vi "TX data interpolation to DRAM.vi"() -> ()   [LabVIEW 2019]
uses:
  SubVIs/DRAM burst sequencer/Burst memo.ctl
  SubVIs/DRAM burst sequencer/DRAM mode.ctl
  SubVIs/DRAM burst sequencer/SegementSequencer_class/FPGA sequencer states.ctl
  <vilib>/Platform/TimedLoop/XDataNode/timing_clust.ctl
  <vilib>/Platform/TimedLoop/XDataNode/nitl_modes.ctl
  <vilib>/Platform/TimedLoop/XDataNode/wakeup.ctl
  SubVIs/DRAM burst sequencer/DRAM resources.ctl
  <instrlib>/_niInstr/Memory/v1/FPGA/DRAM U512/niInstr Memory DRAM U512 v1 FPGA.lvclass
  <instrlib>/_niInstr/Memory/v1/FPGA/BRAM U512/niInstr Memory BRAM U512 v1 FPGA.lvclass
  <instrlib>/_niInstr/Memory/v1/FPGA/DRAM U512/Public/Create.vi
  <instrlib>/_niInstr/Memory/v1/FPGA/BRAM U512/Public/Create.vi
  <vilib>/rvi/DataTransferAndStorage/Container/Common/niFpgaContainerGetUniqueNameForEmu.vi
  <vilib>/rvi/DataTransferAndStorage/Container/Common/niFpgaContainerSetEmuInfo.vi
  <vilib>/rvi/eio/common/nirviEmuReportErrorAndStop.vi
  <vilib>/rvi/Emulation/niFpgaSctlEmulationGetInTimedLoop.vi
  <vilib>/rvi/Emulation/niFpgaEmulationReportErrorSimple.vi
  <vilib>/rvi/Emulation/niFpgaGetClockAttributes.vi
  <vilib>/rvi/Emulation/niFpgaCriticalErrorInLSC.vi
  <vilib>/rvi/Emulation/niFpgaProcessEmulError.vi
  <vilib>/Platform/TimedLoop/XDataNode/XDataNode.xnode
  <vilib>/rvi/LocalResourceManager/LocalResourceManager.xnode
  SubVIs/DRAM burst sequencer/SegementSequencer_class/SegmentSequencer.lvclass
  <instrlib>/_niInstr/Memory/v1/FPGA/DRAM/niInstr Memory DRAM v1 FPGA.lvclass
  <vilib>/Platform/TimedLoop/XDataNode/XDNodeRunTimeDep.lvlib
  SubVIs/DRAM burst sequencer/TX burst sequencer.lvlib
  <instrlib>/_niInstr/Basic Elements/v1/FPGA/niInstr Basic Elements v1 FPGA.lvlib
  <instrlib>/_niInstr/Memory/v1/FPGA/BRAM/niInstr Memory BRAM v1 FPGA.lvclass
panel:
  out "bram.debug ctr":T1
  out "bram.last written addr":u32
  in  "seq.start":bool
  in  "seq.rst":bool
  out "seq.state":T2
  out "seq.step ctr":u32
  out "seq.repeat ctr":u64
  out "seq.loaded steps":u32
  out "seq.req ctr":i64
  in  "seq.continous":bool
  in  "seq.add step":bool
  in  "seq.new step":T3
  in  "memo.reset":bool
  in  "memo.ctr rst":bool
  out "dram.last written addr":u32
  out "dram.debug ctr":T1
  in  "memo mode":T4
  out "flush":bool
  in  "iq.load":bool
  in  "iq.load addr":u32
  in  "burst memo":T5
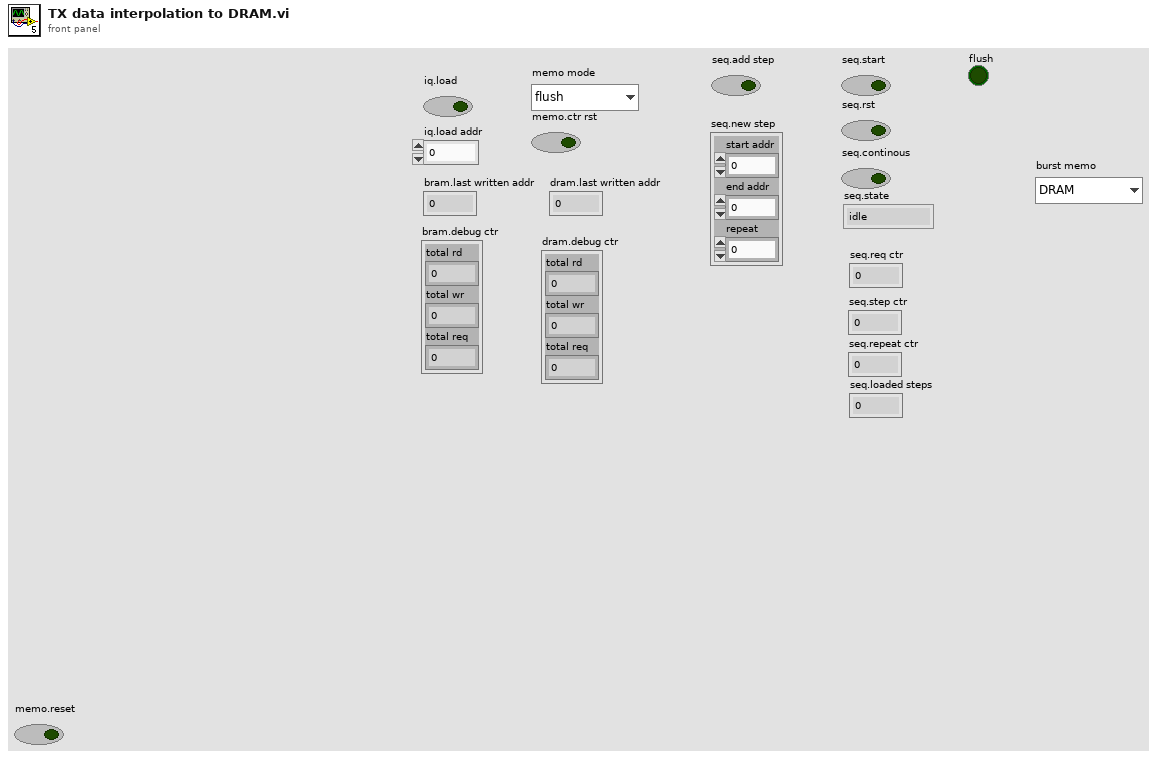
[diagram p1: front panel]
types:
  T1 = cluster{"total rd":u32, "total wr":u32, "total req":u32}
  T2 = typedef "FPGA sequencer states.ctl" = enum16{"idle", "read step", "execute step"}
  T3 = cluster{"start addr":u32, "end addr":u32, "repeat":u64}
  T4 = typedef "TX burst sequencer.lvlib/DRAM mode.ctl" = enum16{"flush", "reset", "write", "read"}
  T5 = typedef "TX burst sequencer.lvlib/Burst memo.ctl" = enum16{"DRAM", "BRAM"}
  T6 = typedef "TX burst sequencer.lvlib/DRAM resources.ctl" = cluster{"DRAM read data FIFO":refnum<k21>, "DRAM write data FIFO":refnum<k21>, "DRAM request FIFO":refnum<k21>, "DRAM U512 memo":refnum<class "niInstr Memory DRAM U512 v1 FPGA.lvclass">, "DMA data loader":refnum<k21>, "BRAM read data FIFO":refnum<k21>, "BRAM write data FIFO":refnum<k21>, "BRAM request FIFO":refnum<k21>, "BRAM U512 memo":refnum<class "niInstr Memory BRAM U512 v1 FPGA.lvclass">}
  T7 = typedef "XDNodeRunTimeDep.lvlib/timing_clust.ctl" = cluster{"Expected End [f-1]":u64, "Actual End [f-1]":u64, "Finished Late? [f-1]":bool, "Expected End [i-1]":u64, "Actual End [i-1]":u64, "Finished Late? [i-1]":bool, "Expected Start [i]":u64, "Actual Start [i]":u64, "Expected Start [f]":u64, "Actual Start [f]":u64, "Source Name":string, "Structure Name":string, "Period":i64, "Deadline":i64, "Offset":i64, "Start":i64, "Priority":i32, "Timeout":i32, "Mode":T8, "Wakeup Reason":T9, "Error":errorcluster, "Source Type":string, "Secondary Source Type":string, "Global End Time":u64, "Global Start Time":u64, "Frame Duration":u64, "Iteration Duration":u64, "Assigned CPU":i32, "I/O Scan Engine Mode":u32}
  T8 = typedef "XDNodeRunTimeDep.lvlib/nitl_modes.ctl" = enum32{"No Change", "Process missed periods, maintain original phase", "Discard missed periods, maintain original phase", "Process missed periods, ignore original phase", "Discard missed periods, ignore original phase"}
  T9 = typedef "XDNodeRunTimeDep.lvlib/wakeup.ctl" = enum32{"Normal", "Aborted", "Asynchronous wakeup", "Timing source error", "Timed loop error", "Timeout"}
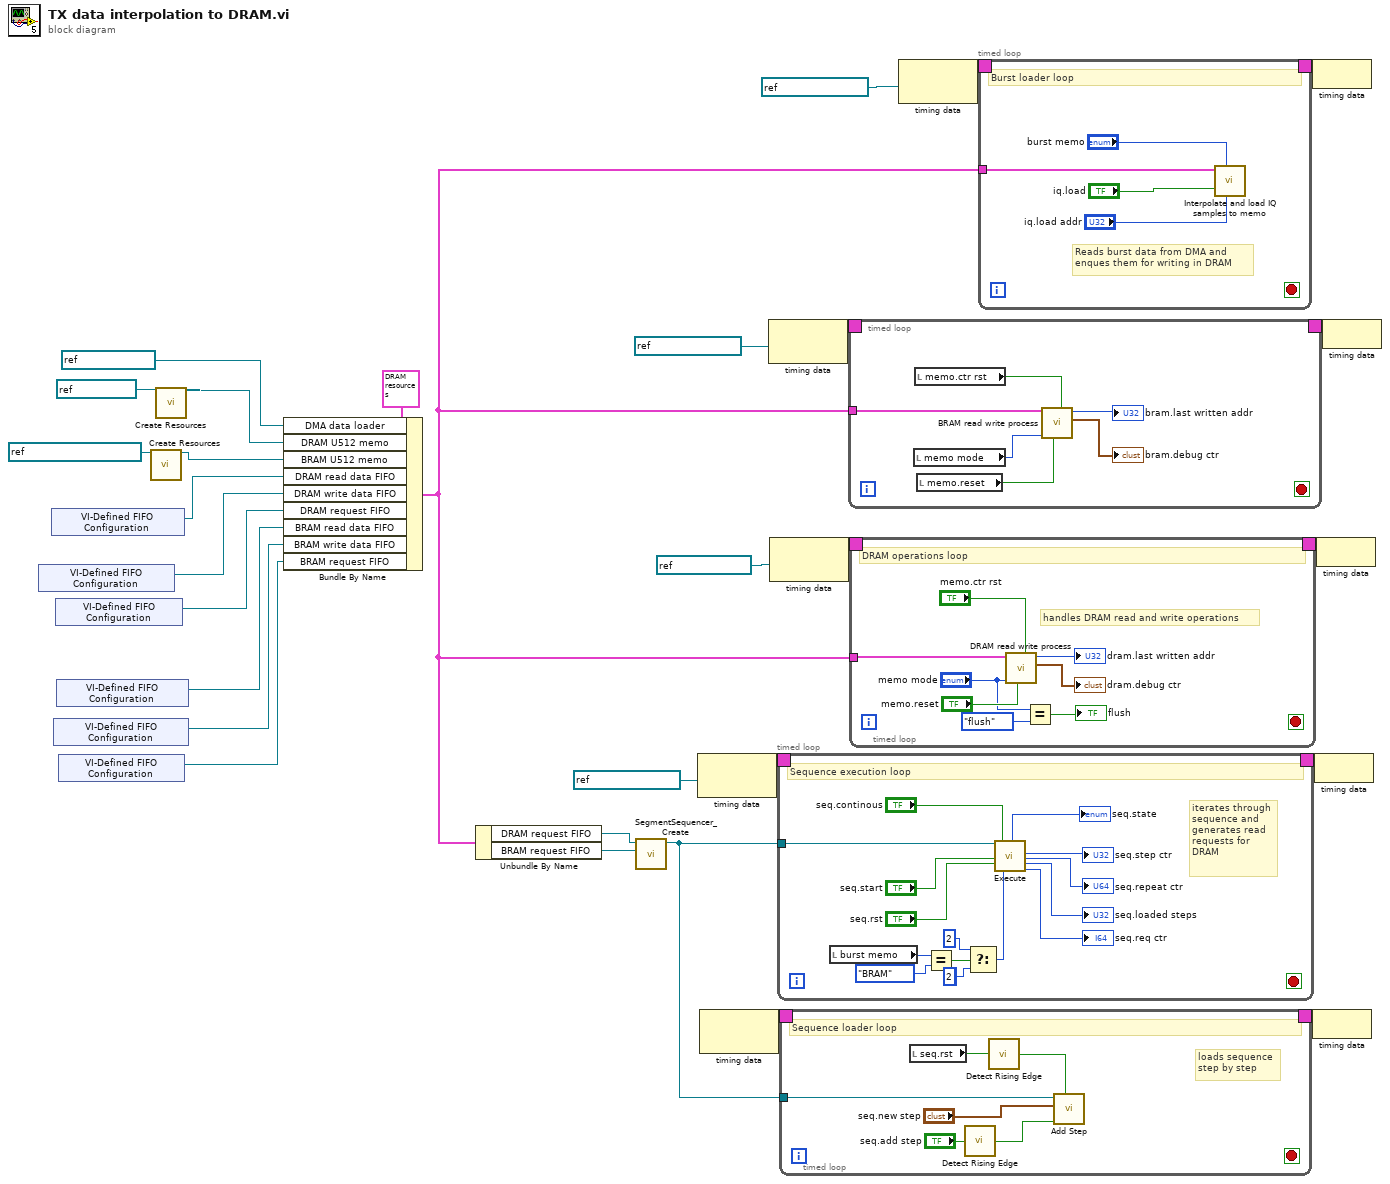
[diagram p0: block diagram]
diagram:
  n1 = xnode "VI-Defined FIFO Configuration"() -> ("FIFO Out"=w17:refnum<k21>)
  n2 = xnode "VI-Defined FIFO Configuration"() -> ("FIFO Out"=w18:refnum<k21>)
  n3 = xnode "VI-Defined FIFO Configuration"() -> ("FIFO Out"=w9:refnum<k21>)
  n4 = xnode "VI-Defined FIFO Configuration"() -> ("FIFO Out"=w16:refnum<k21>)
  n5 = xnode "VI-Defined FIFO Configuration"() -> ("FIFO Out"=w10:refnum<k21>)
  n6 = xnode "VI-Defined FIFO Configuration"() -> ("FIFO Out"=w8:refnum<k21>)
  n7 = call-poly <instrlib>:"Create Resources.vi"("memory in"=refnum<k21> "generation memory") -> ("memory out"=w2:refnum<class "niInstr Memory BRAM U512 v1 FPGA.lvclass">)  [unwired: 14 in]
  n8 = call-poly <instrlib>:"Create Resources.vi"("memory in"=refnum<k21> "TX memo") -> ("memory out"=w15:refnum<class "niInstr Memory DRAM U512 v1 FPGA.lvclass">)  [unwired: 14 in]
  n9 = Bundle By Name(cluster=T6 {"DRAM read data FIFO"="", "DRAM write data FIFO"="", "DRAM request FIFO"="", "DRAM U512 memo"=refnum, "DMA data loader"="custom data", "BRAM read data FIFO"="", "BRAM write data FIFO"="", "BRAM request FIFO"="", "BRAM U512 memo"=refnum} ("DRAM resources"), "DMA data loader"=refnum<k21> "custom data" ("FIFO In"), "DRAM U512 memo"=w15, "BRAM U512 memo"=w2, "DRAM read data FIFO"=w18, "DRAM write data FIFO"=w17, "DRAM request FIFO"=w16, "BRAM read data FIFO"=w10, "BRAM write data FIFO"=w9, "BRAM request FIFO"=w8) -> (w4:T6)
  n10 = Unbundle By Name(w4) -> ("DRAM request FIFO"=w6:refnum<k21>, "BRAM request FIFO"=w5:refnum<k21>)
  n11 = call "SegmentSequencer_Create.vi"("req fifo 2"=w5, "req fifo 1"=w6) -> ("New SegmentSequencer"=w11:refnum<class "SegmentSequencer.lvclass">)  [unwired: 9 in]
  n12 = node-c288(refnum<k21> "200 MHz Clock" ("Source Name")) -> (w24:T7)
  n13 = node-c288() -> (w26:T7)  [unwired: 1 in]
  n14 = node-c288(refnum<k21> "200 MHz Clock" ("Source Name")) -> (w22:T7)
  n15 = node-c288(refnum<k21> "DRAM Clock" ("Source Name")) -> (w28:T7)
  n16 = timed-loop {
    timing: w24 -> [_]
    timing-out: [_] -> w23
    tunnel: w11 -> [w39]
    stop <- _ stop-if-true
    (unwired) i16 2 ("req fifo")
    # "iterates through\nsequence and\ngenerates read\nrequests for\nDRAM"
    # "Sequence execution loop"
    n17 = local read "burst memo"() -> (w36:T5)
    n18 = Equal?(x=w36, y=Burst_memo."BRAM") -> (x = y?=w34:bool)
    n19 = Select(t=i16 2 ("req fifo"), s=w34, f=i16 1 ("req fifo")) -> (s? t:f=w31:i16)
    n20 = call-dynamic "Execute.vi"("SegmentSequencer in"=w39, "start"="seq.start", "reset"="seq.rst", "continuous?"="seq.continous", "req fifo"=w31) -> ("state"=→"seq.state":T2, "step counter"=→"seq.step ctr":u32, "repeat counter"=→"seq.repeat ctr":u64, "Loaded steps"=→"seq.loaded steps":u32, "generated requests"=→"seq.req ctr":i64)  [unwired: 9 in, 1 out]
  }
  n21 = timed-loop {
    timing: w26 -> [_]
    timing-out: [_] -> w25
    tunnel: w11 -> [w53]
    stop <- _ stop-if-true
    # "loads sequence\nstep by step"
    # "Sequence loader loop"
    n22 = local read "seq.rst"() -> (w49:bool)
    n23 = call <instrlib>:"Detect Rising Edge.vi"("signal"="seq.add step") -> ("edge detected"=w52:bool)  [unwired: 14 in]
    n24 = call <instrlib>:"Detect Rising Edge.vi"("signal"=w49) -> ("edge detected"=w48:bool)  [unwired: 14 in]
    n25 = call-dynamic "Add Step.vi"("reset load"=w48, "input valid"=w52, "Data"="seq.new step", "SegmentSequencer in"=w53) -> ()  [unwired: 7 in, 1 out]
  }
  n26 = timed-loop {
    timing: w22 -> [_]
    timing-out: [_] -> w21
    tunnel: w4 -> [w61]
    stop <- _ stop-if-true
    n27 = local read "memo mode"() -> (w60:T4)
    n28 = local read "memo.ctr rst"() -> (w58:bool)
    n29 = local read "memo.reset"() -> (w59:bool)
    n30 = call "BRAM read write process.vi"("debug ctr reset"=w58, "dram.reset"=w59, "dram mode"=w60, "DRAM resources"=w61) -> ("BRAM debug ctr"=→"bram.debug ctr":T1, "last written addr"=→"bram.last written addr":u32)  [unwired: 6 in]
  }
  n31 = timed-loop {
    timing: w28 -> [_]
    timing-out: [_] -> w27
    tunnel: w4 -> [w67]
    stop <- _ stop-if-true
    # "handles DRAM read and write operations"
    # "DRAM operations loop"
    n32 = call "DRAM read write process.vi"("debug ctr reset"="memo.ctr rst", "dram.reset"="memo.reset", "dram mode"="memo mode", "DRAM resources"=w67) -> ("DRAM debug ctr"=→"dram.debug ctr":T1, "last written addr"=→"dram.last written addr":u32)  [unwired: 6 in]
    n33 = Equal?(x="memo mode", y=DRAM_mode."flush") -> (x = y?=→"flush":bool)
  }
  n34 = node-c288(refnum<k21> "100 MHz Clock" ("Source Name")) -> (w30:T7)
  n35 = timed-loop {
    timing: w30 -> [_]
    timing-out: [_] -> w29
    tunnel: w4 -> [w77]
    stop <- _ stop-if-true
    # "Reads burst data from DMA and\nenques them for writing in DRAM"
    # "Burst loader loop"
    n36 = call "Interpolate and load IQ samples to memo.vi"("wr.start addr"="iq.load addr", "burst memo"="burst memo", "wr.enable"="iq.load", "DRAM resources"=w77) -> ()  [unwired: 8 in]
  }
  n37 = node-c288(w29) -> ()
  n38 = node-c288(w25) -> ()
  n39 = node-c288(w23) -> ()
  n40 = node-c288(w27) -> ()
  n41 = node-c288(w21) -> ()
